vi "PP.Create.1x1.BlackPNG.vi"(8 "error in":errorcluster, 11 "file path (use dialog)":path) -> (0 "error out":errorcluster, 3 "file path out":path)   [LabVIEW 2020, in "PixPack.lvlib"]
uses:
  PixPack.lvlib
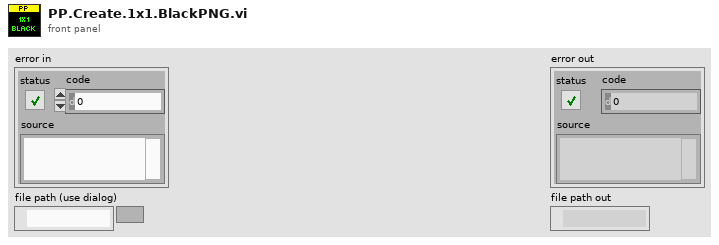
[diagram p1: front panel]
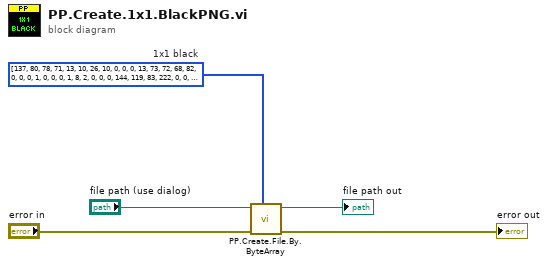
[diagram p0: block diagram]
diagram:
  w5 = u8[] [137, 80, 78, 71, 13, 10, 26, 10, 0, 0, 0, 13, 73, 72, 68, 82, 0, 0, 0, 1, 0, 0, 0, 1, 8, 2, 0, 0, 0, 144, 119, 83, 222, 0, 0, 0, 10, 73, 68, 65, 84, 120, 156, 99, 96, 0, 0, 0, 2, 0, 1, 5, 223, 2, 45, 0, 0, 0, 0, 73, 69, 78, 68, 174, 66, 96, 130]  # 1x1 black
  n1 = call "PP.Create.File.By.ByteArray.vi"("u8 Data[]"=w5, "error in"="error in", "file path (use dialog)"="file path (use dialog)") -> ("error out"=→"error out":errorcluster, "file path out"=→"file path out":path)  [unwired: 7 in]
